vi "Homography.v2.vi"() -> ()   [LabVIEW 2015]
uses:
  <vilib>/Analysis/Matrix/Datatypes/RealMatrix.ctl
  <vilib>/Analysis/baseanly.llb/Real A x B.vi
  <vilib>/Analysis/Matrix/Numeric/Conversions/Matrix To Array - RM.vi
  <vilib>/Analysis/baseanly.llb/Real Inverse Matrix.vi
  <vilib>/Analysis/Matrix/Numeric/Conversions/Array To Matrix - RA2.vi
  <vilib>/Analysis/Matrix/Numeric/Multiply/Multiply - RM,RM.vi
  <vilib>/Analysis/Matrix/NI_Matrix.lvlib
  <vilib>/Analysis/NI_AALBase.lvlib
panel:
  out "output variable":dbl
  out "Array":cluster{"x_out":dbl, "y_out":dbl}[](array[cluster])
  out "XY Graph 2":cluster{dbl, dbl}[](graph)
  out "A x B":T1
  out "XY Graph":cluster{dbl, dbl}[](graph)
  out "appended array":T1
  out "C":T1
  out "B":T1
  out "Factors":T1
  out "Inverse Matrix":T1
  out "Inpu array 2":T1
  out "temp":T1
  out "Input":T1
  in  "y":dbl[][](array[numeric])
  in  "x":dbl[][](array[numeric])
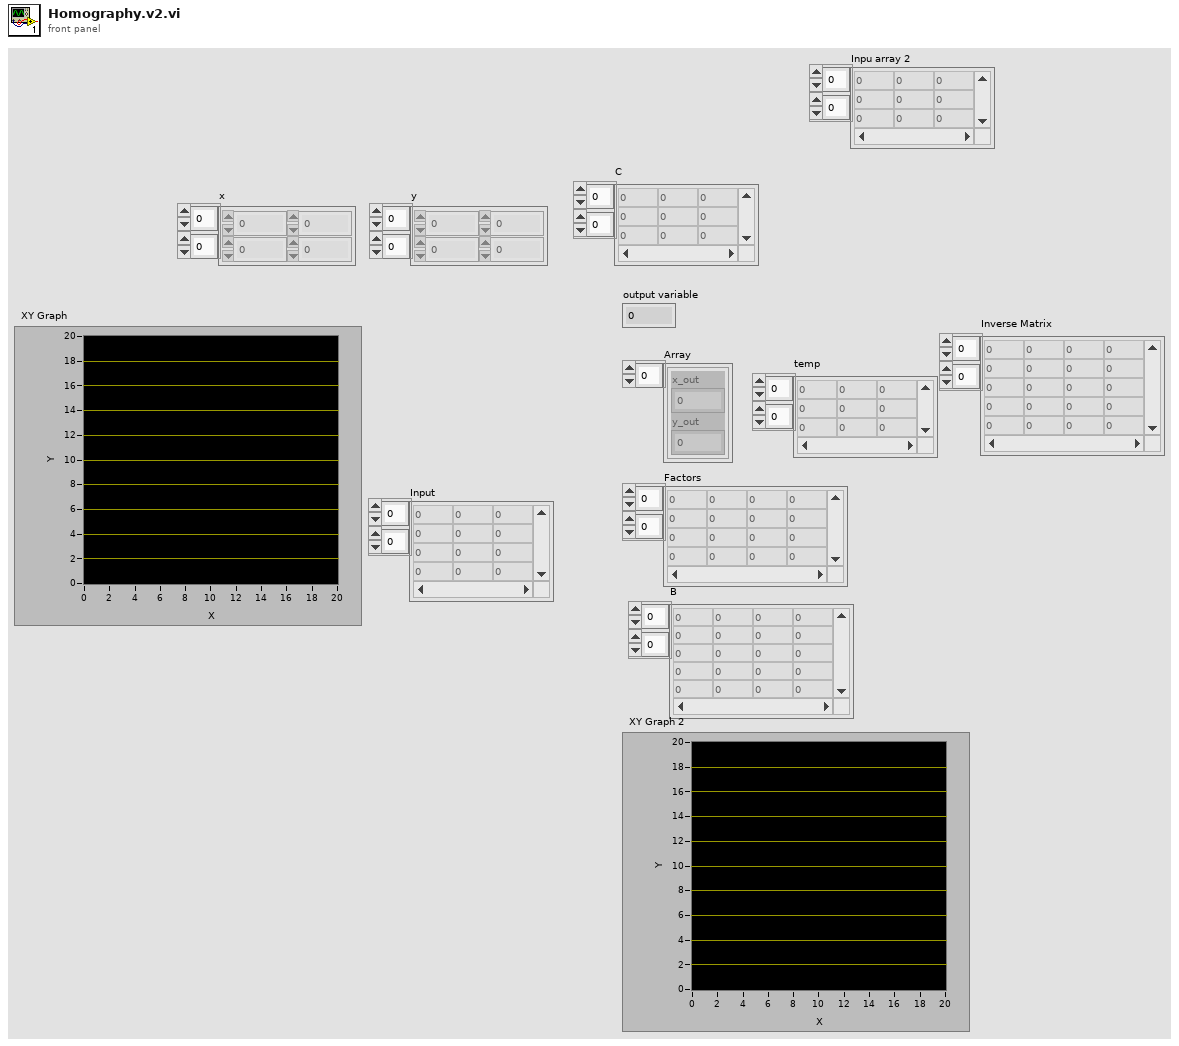
[diagram p1: front panel]
types:
  T1 = typedef "NI_Matrix.lvlib/RealMatrix.ctl" = dbl[][]
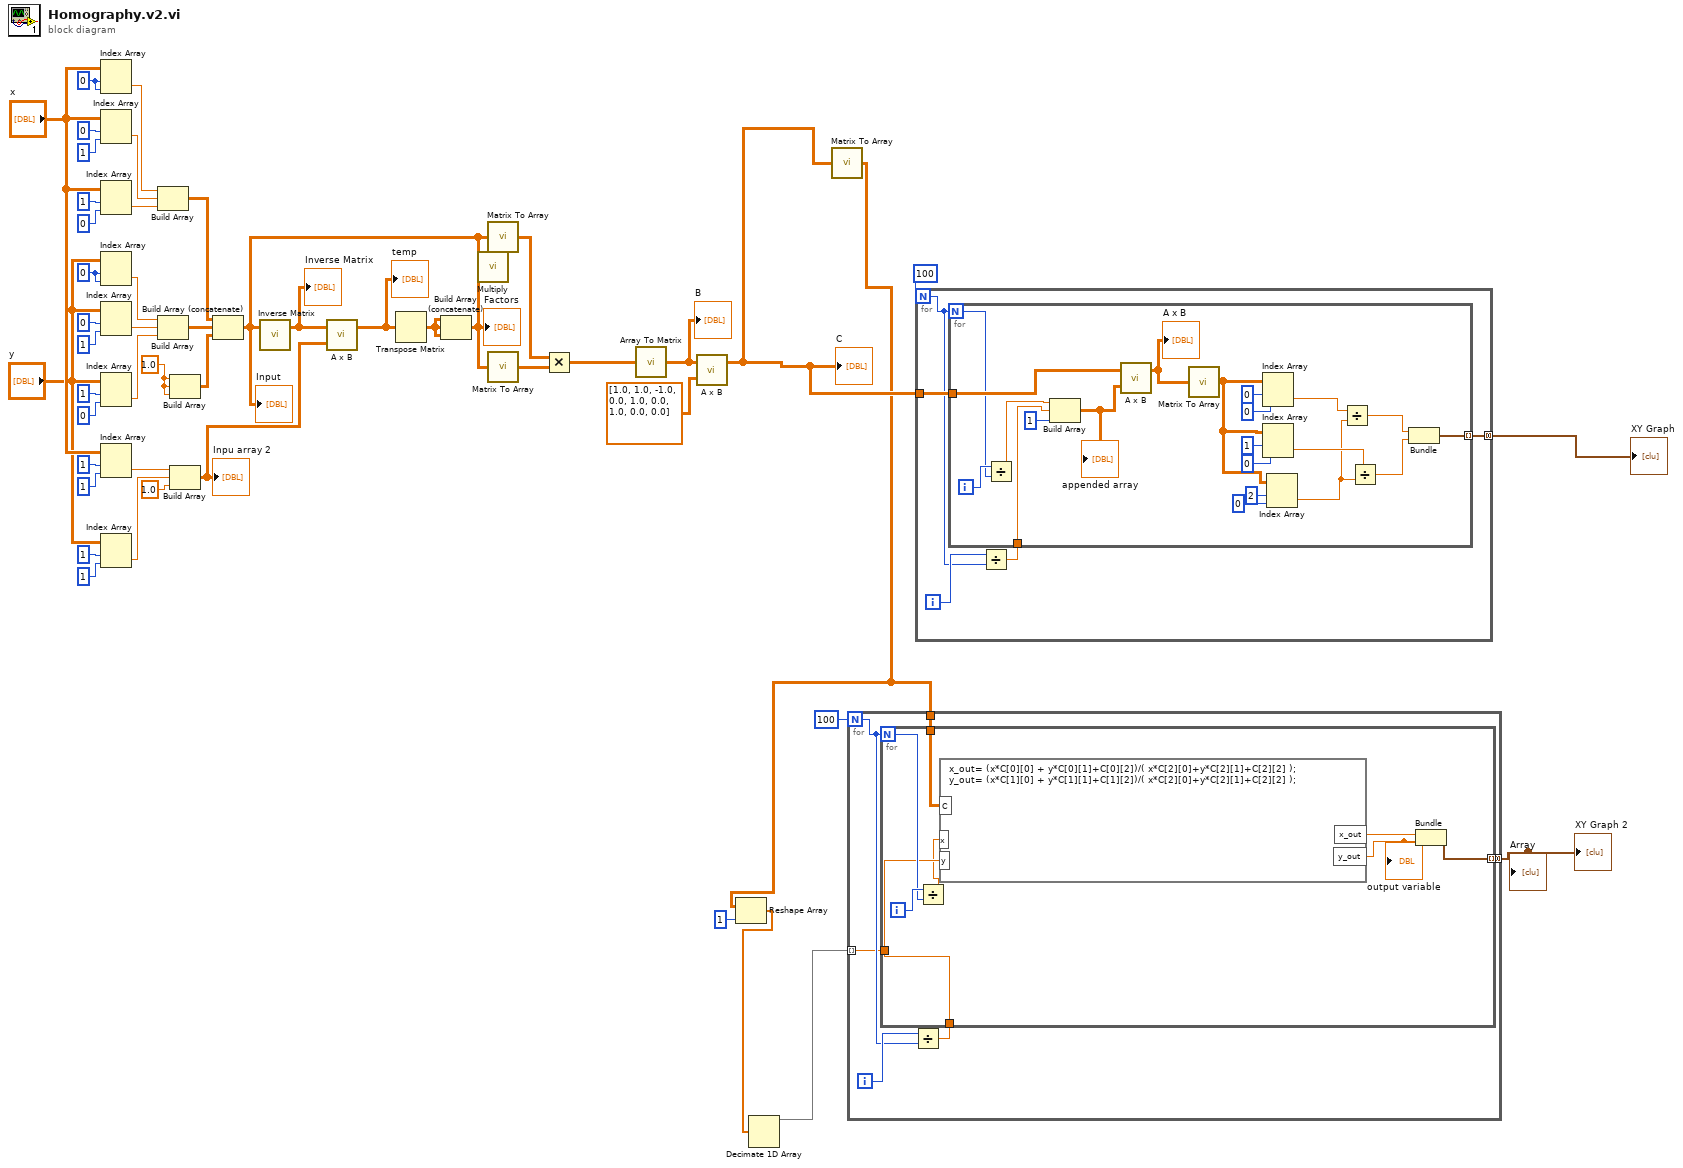
[diagram p0: block diagram]
diagram:
  w35 = 1.0 ("index (row)")
  w39 = 0 ("index (row)")
  w48 = 0 ("index (row)")
  n1 = Index Array(array="x", index (row)=w48, index (col)=w48) -> (element=w49:dbl)
  n2 = Index Array(array="x", index (row)=0 ("index (col)"), index (col)=1) -> (element=w44:dbl)
  n3 = Index Array(array="x", index (row)=1, index (col)=0) -> (element=w43:dbl)
  n4 = Index Array(array="y", index (row)=w39, index (col)=w39) -> (element=w36:dbl)
  n5 = Index Array(array="y", index (row)=0 ("index (col)"), index (col)=1) -> (element=w37:dbl)
  n6 = Index Array(array="y", index (row)=1, index (col)=0) -> (element=w38:dbl)
  n7 = Index Array(array="x", index (row)=1, index (col)=1) -> (element=w25:dbl)
  n8 = Index Array(array="y", index (row)=1, index (col)=1) -> (element=w24:dbl)
  n9 = Build Array(w49, w44, w43) -> (w34:T1)
  n10 = Build Array(w36, w37, w38) -> (w33:T1)
  n11 = Build Array(w35, w35, w35) -> (w32:T1)
  n12 = Build Array(w25, w24, 1.0 ("index (row)")) -> (w22:T1)
  "Inpu array 2" <- w22
  n13 = Build Array (concatenate)(w34, w33, w32) -> (w16:T1)
  "Input" <- w16
  n14 = call-poly <vilib>:"Inverse Matrix.vi"("Input Matrix"=w16) -> ("Inverse Matrix"=w17:T1)  [unwired: 1 in, 1 out]
  "Inverse Matrix" <- w17
  n15 = call-poly <vilib>:"A x B.vi"("B"=w22, "A"=w17) -> ("A x B"=w19:T1)  [unwired: 1 out]
  "temp" <- w19
  n16 = Transpose Matrix(1:w19) -> (0:w18:T1)
  n17 = Build Array (concatenate)(w18, w18, w18) -> (w12:T1)
  "Factors" <- w12
  n18 = call-poly <vilib>:"Multiply.vi"("Real Matrix B"=w12, "Real Matrix A"=w16) -> ()  [unwired: 1 out]
  n19 = call-poly <vilib>:"Matrix To Array.vi"("Real Matrix"=w16) -> ("Real 2D Array"=w15:dbl[][])
  n20 = call-poly <vilib>:"Matrix To Array.vi"("Real Matrix"=w12) -> ("Real 2D Array"=w13:dbl[][])
  n21 = Multiply(x=w15, y=w13) -> (x*y=w14:dbl[][])
  n22 = call-poly <vilib>:"Array To Matrix.vi"("Real 2D Array"=w14) -> ("Real Matrix"=w11:T1)
  "B" <- w11
  n23 = call-poly <vilib>:"A x B.vi"("B"=T1 [[1.0, 1.0, -1.0], [0.0, 1.0, 0.0], [1.0, 0.0, 0.0]] ("appended array"), "A"=w11) -> ("A x B"=w9:T1)  [unwired: 1 out]
  "C" <- w9
  n24 = call-poly <vilib>:"Matrix To Array.vi"("Real Matrix"=w9) -> ("Real 2D Array"=w8:dbl[][])
  n25 = Reshape Array(w8, 1 ("dimension size")) -> (w2:dbl[])
  n26 = Decimate 1D Array(w2) -> (w1:dbl[])  [unwired: 3 out]
  n27 = for {
    N: 100 -> [w52]
    tunnel: [w53] -> w4 mode=concatenating
    tunnel: w8 -> [w51]
    tunnel: w1 -> [w50] mode=indexing
    i -> [w55]
    n28 = Divide(x=w55, y=w52) -> (x/y=w54:dbl)
    n29 = for {
      N: w52 -> [w61]
      tunnel: w54 -> [w57]
      tunnel: [w62] -> w53 mode=indexing
      tunnel: w51 -> [w58]
      tunnel: w50 -> [_]
      i -> [w63]
      n30 = Divide(x=w63, y=w61) -> (x/y=w56:dbl)
      n31 = formula code="x_out= (x*C[0][0] + y*C[0][1]+C[0][2])/( x*C[2][0]+y*C[2][1]+C[2][2] );\ny_out= (x*C[1][0] + y*C[1][1]+C[1][2])/( x*C[2][0]+y*C[2][1]+C[2][2] );"("C"=w58, "x"=w56, "y"=w57) -> ("x_out"=w60:dbl, "y_out"=w59:dbl)
      "output variable" <- w59
      n32 = Bundle("x_out"=w60, "y_out"=w59) -> (w62:cluster{"x_out":dbl, "y_out":dbl})  [unwired: 1 in]
    }
  }
  "XY Graph 2" <- w4
  "Array" <- w4
  n33 = for {
    N: 100 ("y") -> [w64]
    tunnel: w9 -> [w68]
    tunnel: [w65] -> w6 mode=concatenating
    i -> [w67]
    n34 = Divide(x=w67, y=w64) -> (x/y=w66:dbl)
    n35 = for {
      N: w64 -> [w69]
      tunnel: w68 -> [w84]
      tunnel: w66 -> [w87]
      tunnel: [w70] -> w65 mode=indexing
      i -> [w88]
      n36 = Divide(x=w88, y=w69) -> (x/y=w86:dbl)
      n37 = Build Array(w86, w87, 1 ("index (row)")) -> (w85:T1)
      "appended array" <- w85
      n38 = call-poly <vilib>:"A x B.vi"("B"=w85, "A"=w84) -> ("A x B"=w83:T1)  [unwired: 1 out]
      "A x B" <- w83
      n39 = call-poly <vilib>:"Matrix To Array.vi"("Real Matrix"=w83) -> ("Real 2D Array"=w79:dbl[][])
      n40 = Index Array(array=w79, index (row)=0, index (col)=0 ("disabled index (col)")) -> (element=w75:dbl)
      n41 = Index Array(array=w79, index (row)=1, index (col)=0 ("disabled index (col)")) -> (element=w74:dbl)
      n42 = Index Array(array=w79, index (row)=2, index (col)=0 ("disabled index (col)")) -> (element=w73:dbl)
      n43 = Divide(x=w75, y=w73) -> (x/y=w72:dbl)
      n44 = Divide(x=w74, y=w73) -> (x/y=w71:dbl)
      n45 = Bundle(w72, w71) -> (w70:cluster{dbl, dbl})  [unwired: 1 in]
    }
  }
  "XY Graph" <- w6
